vi "PV HLT5xx Measure.vi"(8 "error in (no error)":errorcluster, 9 "HLT 5xx Measure - Cluster":T1={"Parameter"=5, "Parameter\nread only<->describe"=FALSE, "off<->on"=TRUE, "Trigger 1 in"=1e-09} {"Trigger 1 in" min=1e-09 max=1000.0 step=1e-09 format="%.2e"; "Parameter" items=[" Pressure Gauge (read only)", " Zero", " Measure Standby", " Sniff Flow (read only)", " Leakrate  (read only)", " Leakrate  [mbarl/s] (read only)", " Pressure p1 (read only)", " Pressure p2 (read only)", " Trigger 1", " Gauge Type (read only)", " External Pressure Gauge (read only)"]}, 10 "Adress of unit":u16=1 min=1 max=999 step=1, 11 "VISA session":refnum<visa-resource-name>) -> (0 "error out":errorcluster, 2 "response (data)":string, 3 "dup VISA session":refnum<visa-resource-name>)   [LabVIEW 2016, in "Pfeiffer Vacuum.lvlib"]
doc: "There are 11 parameters available, only one of which can be enabled at a time. \n\n0 - Pressure Gauge (read only) - Para 340\n1 - Zero - Para 651\n2 - Measure Standby - Para 653\n3 - Sniff Flow (read only) - Para 659\n4 - Leakrate (read only) - Para 669\n5 - Leakrate [mbarl/s] (read only) (default) - Para 670\n6 - Pressure p1 (read only) - Para 679\n7 - Pressure p2 (read only) - Para 680\n8 - Trigger 1 - Para 681\n9 - Gauga Type (read only) - Para 738\n10 - External Pressure Gauge (read only) - Para 690\n\nNote: The 2 controls right of this one will set the appropriate values for the selected parameter. Any settings for an parameter that is not selected will be ignored. If a value is out of range, it will be changed to either the upper or the lower limit of the range."
uses:
  Pfeiffer Vacuum.lvlib
  PV HLT5xx Measure - Cluster.ctl
panel:
  # "Zero                          :  off  <-------------------> on \n Measure Standby  :  off  <-------------------> on"
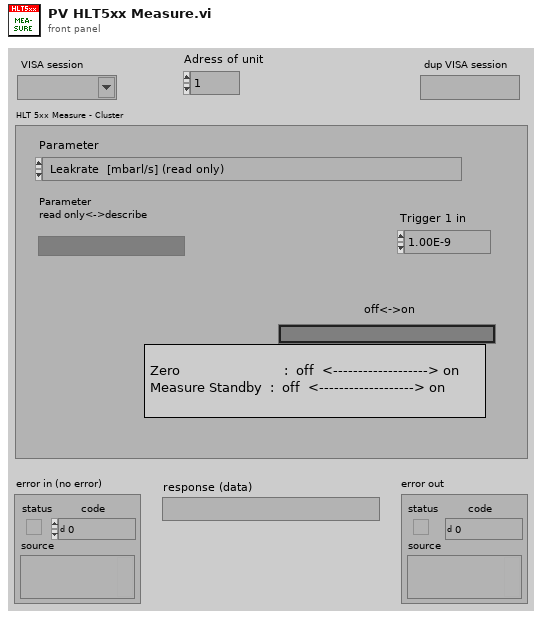
[diagram p1: front panel]
types:
  T1 = typedef "Pfeiffer Vacuum.lvlib/PV HLT5xx Measure - Cluster.ctl" = cluster{"Parameter":u16, "Parameter\nread only<->describe":bool, "off<->on":bool, "Trigger 1 in":dbl}
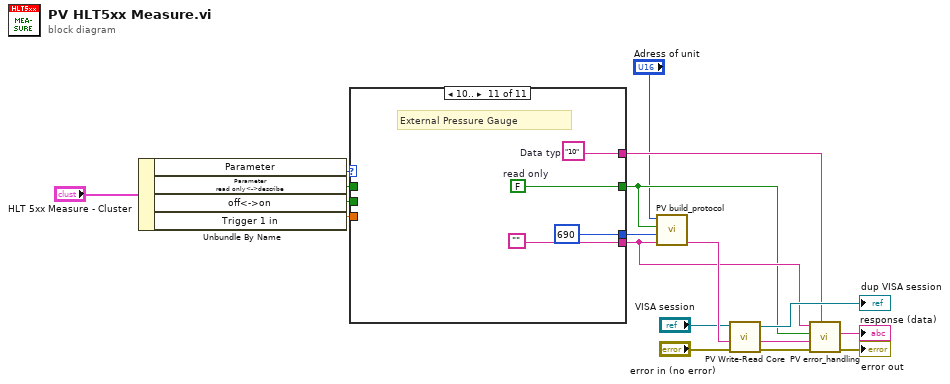
[diagram p0: block diagram]
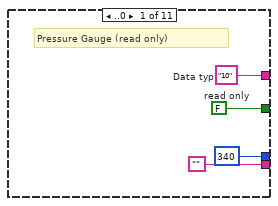
[diagram p2: hidden frame]
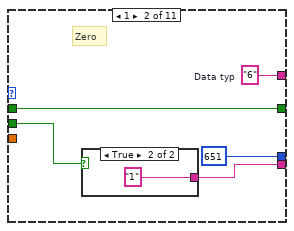
[diagram p3: hidden frame]
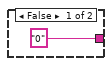
[diagram p4: hidden frame]
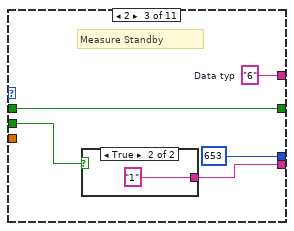
[diagram p5: hidden frame]
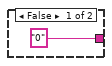
[diagram p6: hidden frame]
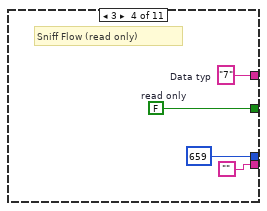
[diagram p7: hidden frame]
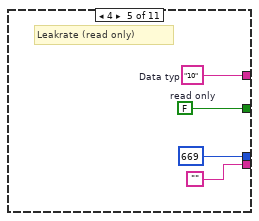
[diagram p8: hidden frame]
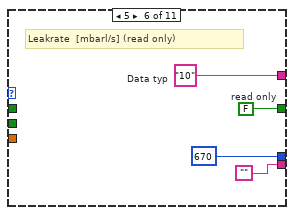
[diagram p9: hidden frame]
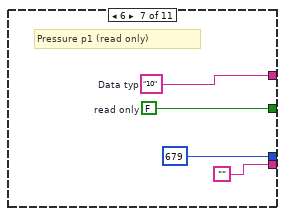
[diagram p10: hidden frame]
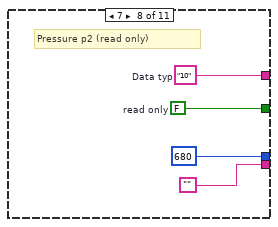
[diagram p11: hidden frame]
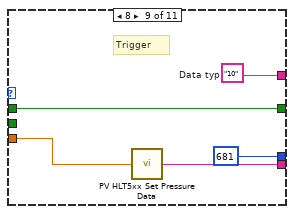
[diagram p12: hidden frame]
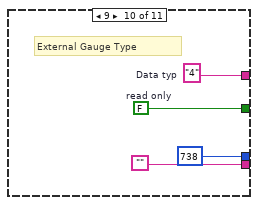
[diagram p13: hidden frame]
diagram:
  n1 = Unbundle By Name("HLT 5xx Measure - Cluster") -> ("Parameter"=w4:u16, "Parameter\nread only<->describe"=w16:bool, "off<->on"=w15:bool, "Trigger 1 in"=w3:dbl)
  n2 = case shown="10.." w4 {
    tunnel: [u16 340 ("Parameter-number") u16 651 ("Parameter-number") u16 653 ("Parameter-number") u16 659 ("Parameter-number") u16 669 ("Parameter-number") u16 670 ("Parameter-number") u16 679 ("Parameter-number") u16 680 ("Parameter-number") u16 681 ("Parameter-number") u16 738 ("Parameter-number") u16 690 ("Parameter-number")] -> w18
    tunnel: ["" w26 w33 "" "" "" "" "" w58 "" ""] -> w11
    tunnel: [w20 w25 w32 w39 w43 w45 w51 w55 w59 w62 w66] -> w9
    tunnel: w16 -> [_ w25 w32 _ _ _ _ _ w59 _ _]
    tunnel: w15 -> [_ w24 w31 _ _ _ _ _ _ _ _]
    tunnel: [w22 w23 w30 w40 w44 w48 w52 w56 w61 w65 w69] -> w10
    tunnel: w3 -> [_ _ _ _ _ _ _ _ w57 _ _]
    frame ..0 {
      w20 = FALSE  # read only
      w22 = "10"  # Data typ
      # "Pressure Gauge (read only)"
    }
    frame 1 {
      w23 = "6"  # Data typ
      # "Zero"
      n3 = case shown="True" w24 {
        tunnel: ["0" ("Data") "1" ("Data")] -> w26
        frame False {
        }
        frame True {
        }
      }
    }
    frame 2 {
      w30 = "6"  # Data typ
      # "Measure Standby"
      n4 = case shown="True" w31 {
        tunnel: ["0" ("Data") "1" ("Data")] -> w33
        frame False {
        }
        frame True {
        }
      }
    }
    frame 3 {
      w39 = FALSE  # read only
      w40 = "7"  # Data typ
      # "Sniff Flow (read only)"
    }
    frame 4 {
      w44 = "10"  # Data typ
      w43 = FALSE  # read only
      # "Leakrate (read only)"
    }
    frame 5 {
      w45 = FALSE  # read only
      w48 = "10"  # Data typ
      # "Leakrate  [mbarl/s] (read only)"
    }
    frame 6 {
      w52 = "10"  # Data typ
      w51 = FALSE  # read only
      # "Pressure p1 (read only)"
    }
    frame 7 {
      w56 = "10"  # Data typ
      w55 = FALSE  # read only
      # "Pressure p2 (read only)"
    }
    frame 8 {
      w61 = "10"  # Data typ
      # "Trigger"
      n5 = call "PV HLT5xx Set Pressure Data.vi"("Value in"=w57) -> ("Output"=w58:string)
    }
    frame 9 {
      w62 = FALSE  # read only
      w65 = "4"  # Data typ
      # "External Gauge Type"
    }
    frame 10.. {
      w66 = FALSE  # read only
      w69 = "10"  # Data typ
      # "External Pressure Gauge"
    }
  }
  n6 = call "PV build_protocol.vi"("Data"=w11, "Parameter-number"=w18, "parameter\nread<->describe"=w9, "Adress"="Adress of unit") -> ("output"=w14:string)  [unwired: 3 in]
  n7 = call "PV Write-Read Core.vi"("error in"="error in (no error)", "Write data in"=w14, "VISA session"="VISA session") -> ("error out"=w13:errorcluster, "response (data) out"=w1:string, "dup VISA session"=→"dup VISA session":refnum<visa-resource-name>)  [unwired: 2 in]
  n8 = call "PV error_handling.vi"("Data Typ in"=w10, "error in"=w13, "response (data) in"=w1, "Parameter\nread only<->describe"=w9, "data in"=w11) -> ("error out"=→"error out":errorcluster, "Data out"=→"response (data)":string)  [unwired: 4 in, 1 out]
